vi "Initialize.vi"(8 "error in (no error)":errorcluster, 11 "Sensor & Control in":refnum<class "Sensor.lvclass">) -> (0 "error out":errorcluster, 3 "Sensor & Control out":refnum<class "Sensor.lvclass">)   [LabVIEW 2013, in "Sensor.lvib.lvlib" / "Sensor.lvclass"]
uses:
  Sensor.lvclass
  Sensor.lvclass/Sensor.ctl
  Read Value.vi
  Read Sampling Interval.vi
  Write VISA.vi
  <vilib>/Instr/_visa.llb/VISA Configure Serial Port (Instr).vi
  PluginInterface/PluginInterface.lvlibp/PluginInterfaceClass/Read Name.vi
  PluginInterface/PluginInterface.lvlibp/PluginInterfaceClass/Read TDMS File Path.vi
  PluginInterface/PluginInterface.lvlibp/PluginInterfaceClass/Read DVR.vi
  PluginInterface/PluginInterface.lvlibp/PluginInterfaceClass/Write TDMS.vi
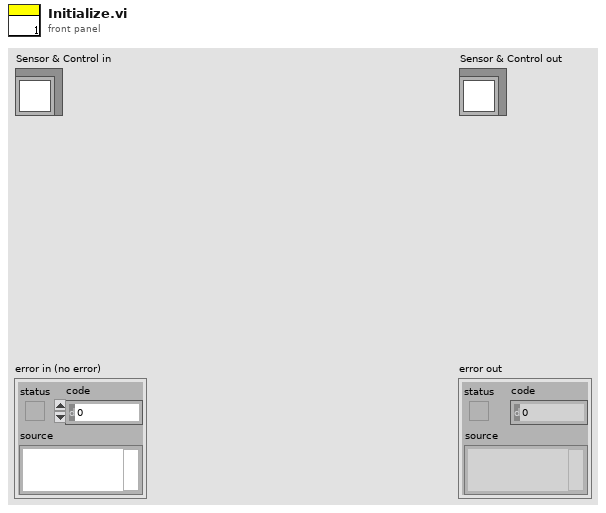
[diagram p1: front panel]
types:
  T1 = enum16{"open", "open or create", "create or replace", "create", "open (read-only)"}
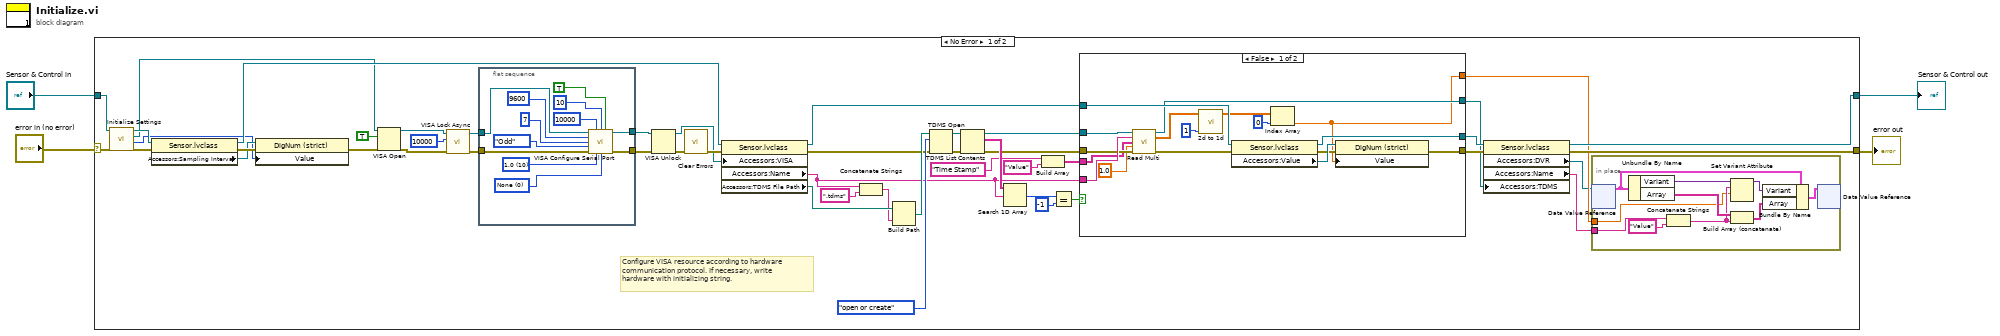
[diagram p0: block diagram]
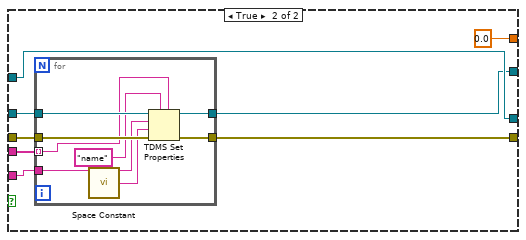
[diagram p2: hidden frame]
diagram:
  n1 = case shown="No Error" "error in (no error)" {
    selector: "error in (no error)" -> [w18 w109]
    tunnel: [w11 w109] -> w3
    tunnel: [w12 w108] -> w1
    tunnel: "Sensor & Control in" -> [w20 w108]
    frame No Error {
      # "Configure VISA resource according to hardware\ncommunication protocol. If necessary, write\nhardware with initializing string."
      n2 = call "Initialize Settings.vi"("error in (no error)"=w18, "Sensor & Control in"=w20) -> ("error out"=w13:errorcluster, "Sampling Interval 2"=w15:i32, "VISA out"=w17:refnum<visa-resource-name>, "Sensor & Control out"=w19:refnum<class "Sensor.lvclass">)  [unwired: 6 in]
      n3 = property class="Sensor.lvclass"(reference=w19, error in=w13) -> (reference out=w22:refnum<class "Sensor.lvclass">, error out=w21:errorcluster, "Accessors:Sampling Interval"=w16:refnum<vi>)
      n4 = property class="DigNum (strict)"(reference=w16, error in=w21, "Value"=w15) -> (error out=w14:errorcluster)  [unwired: 1 out]
      n5 = VISA Open(duplicate session (F)=TRUE, error in (no error)=w14, VISA resource name=w17) -> (VISA resource name=w28:refnum<visa-resource-name>, error out=w31:errorcluster)  [unwired: 2 in]
      n6 = call <vilib>:"VISA Lock Async.vi"("error in (no error)"=w31, "timeout (0)"=u32 10000, "VISA resource name"=w28) -> ("error out"=w30:errorcluster, "VISA resource name out"=w29:refnum<visa-resource-name>)  [unwired: 6 in, 1 out]
      n7 = flat-sequence {
        tunnel: w29 -> [w69]
        tunnel: w30 -> [w68]
        tunnel: [w67] -> w26
        tunnel: [w66] -> w25
        frame #0 {
          w65 = u16 0 items=["None", "XON/XOFF", "RTS/CTS", "XON/XOFF & RTS/CTS", "DTR/DSR", "XON/XOFF & DTR/DSR"] ("flow control (0:none)")
          w71 = u16 10 items=["1.0"=10, "1.5"=15, "2.0"=20] ("stop bits (10: 1 bit)")
          n8 = call-poly "VISA Configure Serial Port"("VISA resource name"=w69, "timeout (10sec)"=u32 10000, "termination char\n(0xA = '\\n' = LF)"=u8 10 ("termination char\n(0xA = '\\n' = LF)"), "Enable Termination\nChar (T)"=TRUE ("Enable Termination\nChar (T)"), "baud rate (9600)"=u32 9600, "data bits (8)"=u16 7, "parity (0:none)"=enum16{"None", "Odd", "Even", "Mark", "Space"}."Odd", "error in (no error)"=w68, "stop bits (10: 1 bit)"=w71, "flow control (0:none)"=w65) -> ("VISA resource name out"=w66:refnum<visa-resource-name>, "error out"=w67:errorcluster)  [unwired: 4 out]
        }
      }
      n9 = VISA Unlock(8:w26, 11:w25) -> (0:w34:errorcluster, 3:w33:refnum<visa-resource-name>)
      n10 = call <vilib>:"Clear Errors.vi"("error in (no error)"=w34) -> ("error out"=w43:errorcluster)  [unwired: 6 in]
      n11 = property class="Sensor.lvclass"(reference=w22, error in=w43, "Accessors:VISA"=w33) -> (reference out=w9:refnum<class "Sensor.lvclass">, error out=w8:errorcluster, "Accessors:Name"=w10:string, "Accessors:TDMS File Path"=w39:path)
      n12 = Concatenate Strings(w10, ".tdms" ("name or relative path")) -> (w23:string)
      n13 = Build Path(base path=w39, name or relative path=w23) -> (appended path=w42:path)
      n14 = TDMS Open(8:w8, 10:T1."open or create" ("operation (0:open)"), 11:w42) -> (0:w41:errorcluster, 3:w38:refnum<k34>)  [unwired: 4 in]
      n15 = TDMS List Contents(4:w41, 7:w38) -> (0:w47:errorcluster, 2:w50:string[], 3:w48:refnum<k34>)  [unwired: 1 in, 1 out]
      n16 = Search 1D Array(1D array=w50, element=w10) -> (index of element=w51:i32)  [unwired: 1 in]
      n17 = Build Array("Time Stamp" ("Channel"), "Value" ("string")) -> (w46:string[])
      n18 = Equal?(x=w51, y=-1) -> (x = y?=w49:bool)
      n19 = case shown="False" w49 {
        tunnel: w48 -> [w86 w99]
        tunnel: [w80 w95] -> w37
        tunnel: w47 -> [w89 w97]
        tunnel: w10 -> [w90 w98]
        tunnel: w9 -> [w91 w94]
        tunnel: w46 -> [w78 w96]
        tunnel: [w85 w94] -> w36
        tunnel: [w77 w93] -> w32
        tunnel: [w75 0.0 ("Numeric Control")] -> w6
        frame False {
          n20 = call "Read Multi.vi"("tdms file in"=w86, "group"=w90, "Channel"=w78, "Numeric"=1.0, "error in (no error)"=w89) -> ("tdms file out"=w77:refnum<k34>, "Array"=w83:dbl[][], "error out"=w88:errorcluster)  [unwired: 7 in, 1 out]
          n21 = call "2d to 1d.vi"("index"=1, "array"=w83) -> ("output array"=w82:dbl[])  [unwired: 9 in]
          n22 = property class="Sensor.lvclass"(reference=w91, error in=w88) -> (reference out=w85:refnum<class "Sensor.lvclass">, error out=w76:errorcluster, "Accessors:Value"=w79:refnum<vi>)
          n23 = Index Array(array=w82, index=0) -> (element=w75:dbl)
          n24 = property class="DigNum (strict)"(reference=w79, error in=w76, "Value"=w75) -> (error out=w80:errorcluster)  [unwired: 1 out]
        }
        frame True {
          n25 = for {
            tunnel: w97 -> [w107]
            tunnel: [w106] -> w95
            tunnel: w99 -> [w105]
            tunnel: w98 -> [w104]
            tunnel: w96 -> [w103] mode=indexing
            tunnel: [w100] -> w93
            n26 = call <vilib>:"Space Constant.vi"() -> ("String"=w101:string)
            n27 = TDMS Set Properties(5:w103, 7:"name" ("property names"), 8:w107, 9:w101, 10:w104, 11:w105) -> (0:w106:errorcluster, 3:w100:refnum<k34>)  [unwired: 2 out]
          }
        }
      }
      n28 = property class="Sensor.lvclass"(reference=w36, error in=w37, "Accessors:TDMS"=w32) -> (reference out=w12:refnum<class "Sensor.lvclass">, error out=w11:errorcluster, "Accessors:DVR"=w5:refnum<data-value>, "Accessors:Name"=w7:string)
      n29 = in-place {
        in-place-border: w6 -> [w53]
        in-place-border: w7 -> [w57]
        n30 = in-place-dvr #1(w5) -> (w59:cluster{"Array":string[], "Variant":variant})  [unwired: 1 out]
        n31 = Unbundle By Name(w59) -> ("Variant"=w61:variant, "Array"=w56:string[])
        n32 = Concatenate Strings(w57, "Value" ("string")) -> (w54:string)
        n33 = Set Variant Attribute(Variant=w61, name=w54, value=w53) -> (Variant out=w60:variant)  [unwired: 1 in, 2 out]
        n34 = Build Array (concatenate)(w56, w54) -> (w55:string[])
        n35 = Bundle By Name(cluster=w59, "Variant"=w60, "Array"=w55) -> (w62:cluster{"Array":string[], "Variant":variant})
        n36 = in-place-dvr #1(w62) -> ()  [unwired: 2 out]
      }
    }
    frame Error {
    }
  }
  "error out" <- w3
  "Sensor & Control out" <- w1
